vi "geracao_onda_senoidal.vi"() -> ()   [LabVIEW 2020]
panel:
  in  "stop":bool
  in  "Amostras/Ciclo":dbl
  # "Geracão de uma onda senoidal pelo número de amostras"
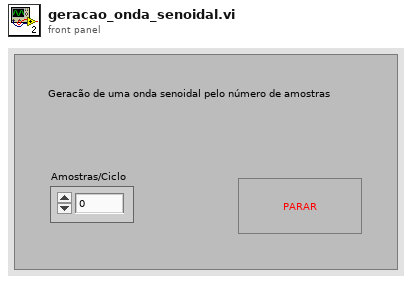
[diagram p1: front panel]
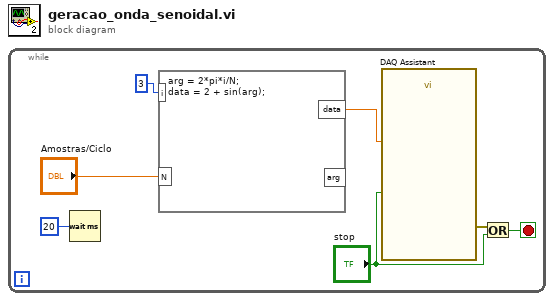
[diagram p0: block diagram]
diagram:
  n1 = while {
    stop <- w6 stop-if-true
    n2 = Wait (ms)(milliseconds to wait=u32 20) -> ()  [unwired: 1 out]
    n3 = formula code="arg = 2*pi*i/N;\ndata = 2 + sin(arg);"("N"="Amostras/Ciclo", "i"=3) -> ("data"=w3:dbl)  [unwired: 1 out]
    n4 = call "DAQ Assistant"("data"=w3, "stop (T)"="stop") -> ("error out"=w5:errorcluster)  [unwired: 16 in, 1 out]
    n5 = Or(x=w5, y="stop") -> (x .or. y?=w6:bool)
  }
